vi "Graphics-Add Plot.vi"(0 "XYGraph in":refnum<vi>, 1 "Name":string, 7 "XY Data":cluster{dbl[], dbl[]}, 9 "Color":u32=4294967295 format="%08x", 11 "error in (no error)":errorcluster, 12 "Plot.Line Width":u8=1, 13 "Plot.Line Style":u8) -> (4 "XYGraph out":refnum<vi>, 15 "error out":errorcluster)   [LabVIEW 2020]
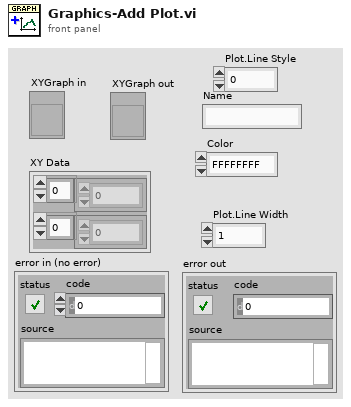
[diagram p1: front panel]
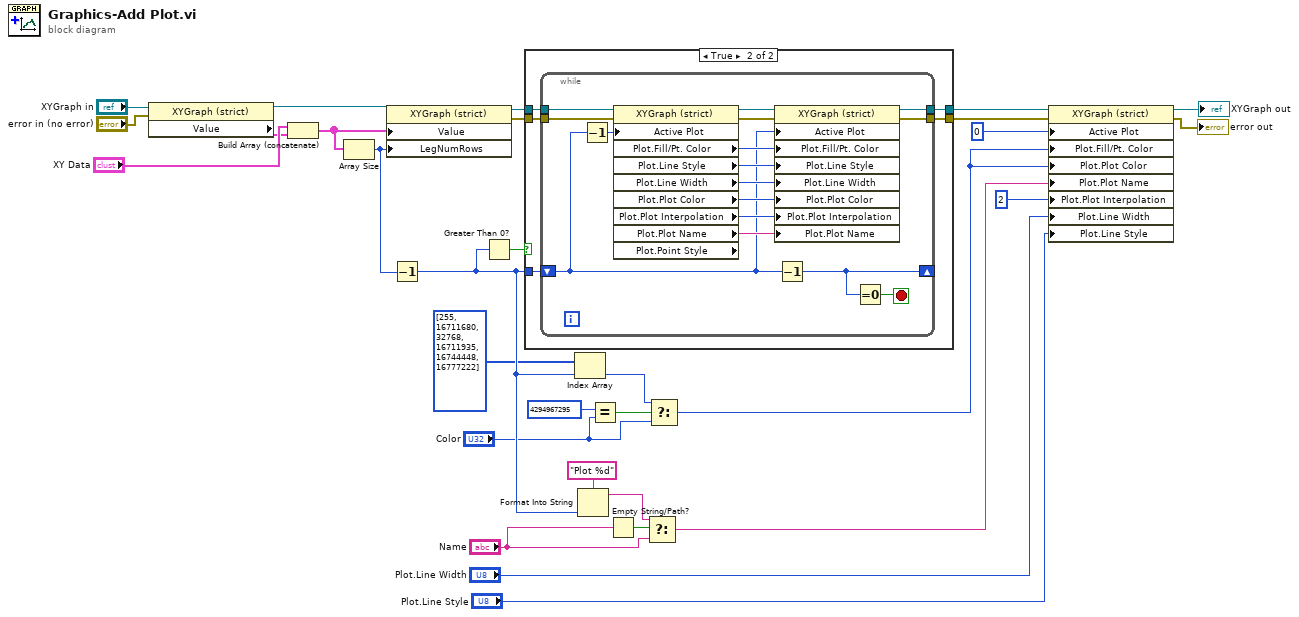
[diagram p0: block diagram]
diagram:
  n1 = property class="XYGraph (strict)"(reference="XYGraph in", error in="error in (no error)") -> (reference out=w29:refnum<vi>, "Value"=w27:cluster{"Frequency":dbl[], "Frequency":dbl[]}[])  [unwired: 1 out]
  n2 = Build Array (concatenate)("XY Data", w27) -> (w30:cluster{"Frequency":dbl[], "Frequency":dbl[]}[])
  n3 = Array Size(array=w30) -> (size(s)=w24:i32)
  n4 = property class="XYGraph (strict)"(reference=w29, "Value"=w30, "LegNumRows"=w24) -> (reference out=w23:refnum<vi>, error out=w22:errorcluster)  [unwired: 1 in]
  n5 = Decrement(x=w24) -> (x-1=w14:i32)
  n6 = Greater Than 0?(x=w14) -> (x > 0?=w15:bool)
  n7 = case shown="True" w15 {
    tunnel: w23 -> [w32 w37]
    tunnel: w22 -> [w31 w36]
    tunnel: [w32 w35] -> w21
    tunnel: [w31 w34] -> w20
    tunnel: w14 -> [_ w33]
    frame False {
    }
    frame True {
      n8 = while {
        shift-right: [w42] -> _
        shift-left: w33 -> [w43]
        tunnel: w37 -> [w38]
        tunnel: w36 -> [w53]
        tunnel: [w40] -> w35
        tunnel: [w39] -> w34
        stop <- w41 stop-if-true
        n9 = Decrement(x=w43) -> (x-1=w52:i32)
        n10 = property class="XYGraph (strict)" props=["Active Plot", "Plot", "Fill/Pt. Color", "Plot", "Line Style", "Plot", "Line Width", "Plot", "Plot Color", "Plot", "Plot Interpolation", "Plot", "Plot Name", "Plot", "Point Style"](reference=w38, error in=w53, "Active Plot"=w52) -> (reference out=w51:refnum<vi>, error out=w50:errorcluster, "Plot.Fill/Pt. Color"=w49:u32, "Plot.Line Style"=w48:u8, "Plot.Line Width"=w47:u8, "Plot.Plot Color"=w46:u32, "Plot.Plot Interpolation"=w45:u8, "Plot.Plot Name"=w44:string)  [unwired: 1 out]
        n11 = property class="XYGraph (strict)"(reference=w51, error in=w50, "Active Plot"=w43, "Plot.Fill/Pt. Color"=w49, "Plot.Line Style"=w48, "Plot.Line Width"=w47, "Plot.Plot Color"=w46, "Plot.Plot Interpolation"=w45, "Plot.Plot Name"=w44) -> (reference out=w40:refnum<vi>, error out=w39:errorcluster)
        n12 = Decrement(x=w43) -> (x-1=w42:i32)
        n13 = Equal To 0?(x=w42) -> (x = 0?=w41:bool)
      }
    }
  }
  n14 = Index Array(array=u32[] [255, 16711680, 32768, 16711935, 16744448, 16777222] ("Color Order"), index=w14) -> (element=w3:u32)
  n15 = Format Into String(format string="Plot %d", w14) -> (resulting string=w10:string)  [unwired: 2 in, 1 out]
  n16 = Equal?(x=u32 4294967295 ("Color 2"), y="Color") -> (x = y?=w5:bool)
  n17 = Empty String/Path?(string/path="Name") -> (empty?=w12:bool)
  n18 = Select(t=w10, s=w12, f="Name") -> (s? t:f=w9:string)
  n19 = Select(t=w3, s=w5, f="Color") -> (s? t:f=w2:u32)
  n20 = property class="XYGraph (strict)"(reference=w21, error in=w20, "Active Plot"=u32 0, "Plot.Fill/Pt. Color"=w2, "Plot.Plot Color"=w2, "Plot.Plot Name"=w9, "Plot.Plot Interpolation"=u8 2, "Plot.Line Width"="Plot.Line Width", "Plot.Line Style"="Plot.Line Style") -> (reference out=→"XYGraph out":refnum<vi>, error out=→"error out":errorcluster)
